vi "Audio Test.Calculate Freq Response.vi"(6 "Sweep Attribues":T1={"ReSampl Times(s)"=array[167426 elements], "Meas Phases (rad)"=[36.81553890925539, 8354.100868622301, 14959.386062088855, 20206.61147531608, 24374.996904709846, 27686.354004414785, 30316.88948878321, 32406.58165059181, 34066.62894449532, 35385.36721306204, 36432.970271774815, 37265.1840554823, 37926.29303158248, 38451.476685983085, 38868.681536741446, 39200.10824052903, 39463.39295419466, 39672.5458075507, 39838.69641775387, 39970.68613219857, 40075.5384988172, 40158.83301016359, 40225.00200445678, 40277.566521725035, 40319.32366977219, 40352.49546510379, 40378.84707330696, 40399.780738497255], "Meas Freqs (Hz)"=[20000.0, 15887.960215532483, 12621.363990517146, 10026.386447354535, 7964.941449056137, 6327.333643082476, 5026.421259584723, 3992.979049939437, 3172.0146143446227, 2519.8420997897483, 2001.7575515441654, 1590.1922170037706, 1263.2455339402636, 1003.5197392845996, 797.1940846627623, 633.28939505899, 503.08383568079324, 399.6487983186957, 317.48021039364005, 252.20564759765148, 200.35166475820458, 159.15896393970277, 126.4355643509683, 100.44016081182906, 79.78946395100115, 63.384591443608464, 50.35259335669159, 40.0], "Samples/rev"=26}, 8 "error in":errorcluster, 9 "Sine Sweep Params":T2={"Duration(s)"=2.0, "Amplitude"=1.0, "Freq Start"=20.0, "Freq End"=20000.0, "Samples/Sec"=44100.0} {"Amplitude" min=0.0 max=1.0 step=0.1}) -> (0 "error out":errorcluster, 2 "THD":cluster{"frequency":dbl[], "THD":dbl[]}(graph), 3 "Magnitude":cluster{"frequency":dbl[], "magnitude":dbl[]}(graph), 10 "Measured":waveform(dbl)(graph)={"t0"=timestamp(0 s since 1904-01-01), "dt"=2.2675736961451248e-05, "Y"=array[88200 elements]}, 11 "Stimulus":waveform(dbl)(graph)={"t0"=timestamp(0 s since 1904-01-01), "dt"=2.2675736961451248e-05, "Y"=array[88200 elements]})   [LabVIEW 2018]
uses:
  TypeDefs/AudioTest.Config, Sine Sweep Params.ctl
  TypeDefs/AudioTest.Sweep Attributes.ctl
  <vilib>/Utility/error.llb/DialogType.ctl
  <vilib>/addons/_NISVFA/_Shared subVIs/Controls/svc_Window.ctl
  <vilib>/addons/_NISVFA/_Shared subVIs/Common/svc_Get Waveform Subset (Index).vi
  <vilib>/addons/_NISVFA/_Shared subVIs/Common/svc_Get Array Subset (Index).vi
  <vilib>/addons/_NISVFA/_Shared subVIs/Common/svc_Coerce Index and Length.vi
  <vilib>/addons/_NISVFA/_Shared subVIs/Common/svc_Conditional Merge Error.vi
  <vilib>/Waveform/WDTOps.llb/WDT Copy Waveform dt DBL.vi
  <vilib>/measure/maresamp.llb/Align N Waveforms (single shot).vi
  <vilib>/addons/_NISVFA/_Baseband FFT/SVFA FFT Spectrum (Complex) (1 Ch).vi
  <vilib>/addons/Sound and Vibration/svt_Single Tone Measurements/SVT Gain and Phase (Frequency).vi
  <vilib>/addons/Sound and Vibration/svt_Distortion/SVT THD and Harmonic Components (Frequency) (1 Ch).vi
  Program Files (x86)/National Instruments/LabVIEW 2018/examples/Sound and Vibration/SoundVib_Audio Examples.lvlib
  <vilib>/measure/NI_MAPro.lvlib
  <vilib>/addons/Sound and Vibration/svt_Single Tone Measurements/SoundVib_SingleTone.lvlib
  <vilib>/addons/Sound and Vibration/svt_Continuous Swept Sine/SoundVib_ContSweptSine.lvlib
  <vilib>/addons/Sound and Vibration/svt_Distortion/SoundVib_Distortion.lvlib
panel:
  in  "Record":path
  in  "Sweep":path
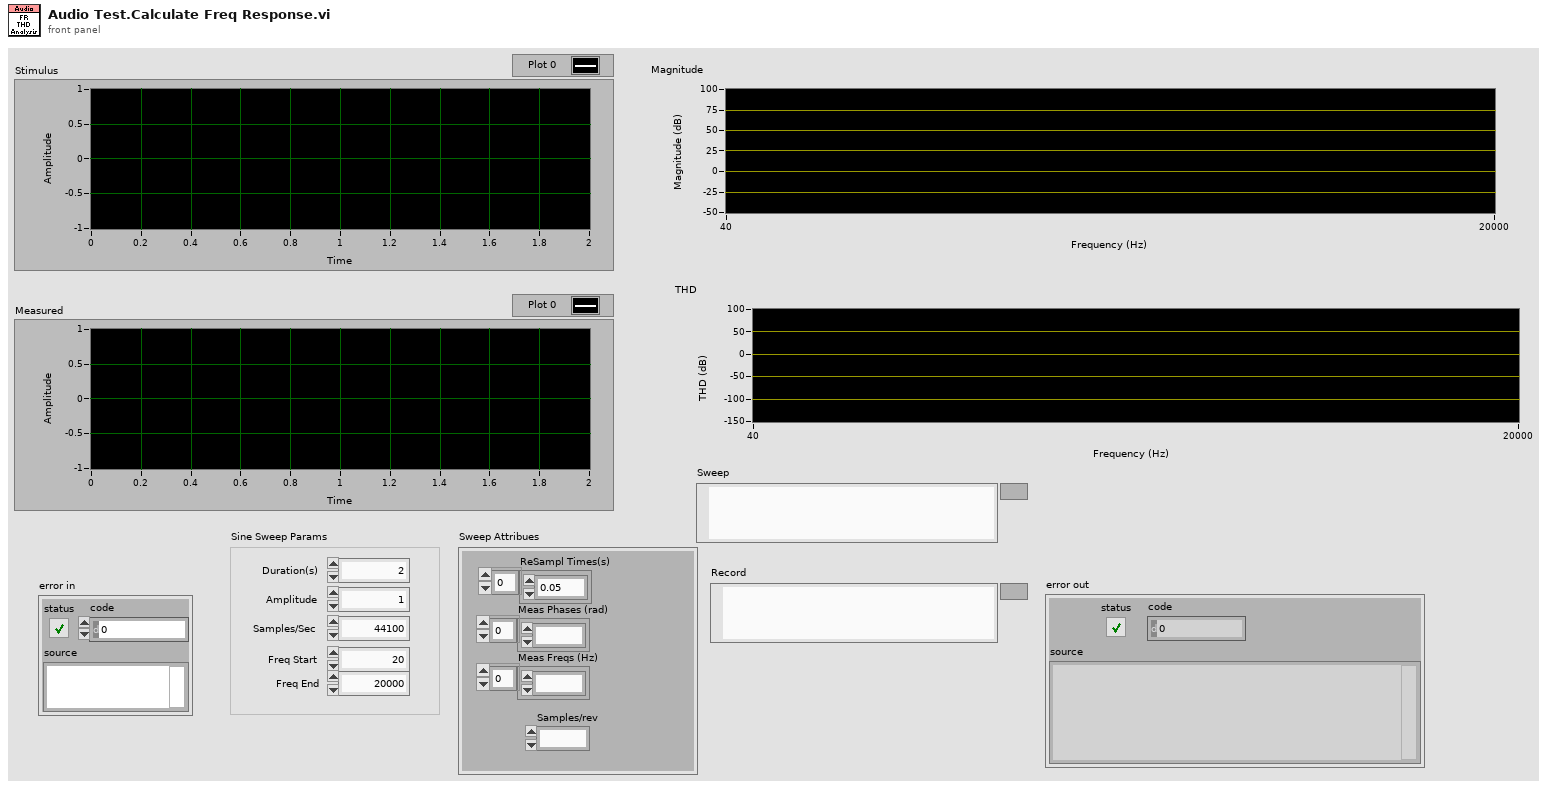
[diagram p1: front panel]
types:
  T1 = typedef "AudioTest.Sweep Attributes.ctl" = cluster{"ReSampl Times(s)":dbl[], "Meas Phases (rad)":dbl[], "Meas Freqs (Hz)":dbl[], "Samples/rev":i32}
  T2 = typedef "AudioTest.Config, Sine Sweep Params.ctl" = cluster{"Duration(s)":dbl, "Amplitude":dbl, "Freq Start":dbl, "Freq End":dbl, "Samples/Sec":dbl}
  T3 = typedef "DialogType.ctl" = u16
  T4 = cluster{"averaging mode":enum16{"No averaging", "Vector averaging", "RMS averaging", "Peak hold"}, "weighting mode":enum16{"Linear", "Exponential"}, "number of averages":u32, "linear mode":enum16{"One shot", "Auto restart"}}
  T5 = typedef "svc_Window.ctl" = u32
  T6 = typedef "svc_Spectrum Info.ctl" = cluster{"channel name":string, "description":string, "x-axis units":T7, "spectral info":cluster{"spectrum type":T8, "linear/dB":enum16{"linear", "dB"}, "window":u16, "window size":i32, "FFT size":i32}, "engineering units":T9, "custom label":string, "dB reference [EU]":dbl, "peak units":enum16{"rms", "peak", "peak-peak"}, "weighting filter":T10, "spectral density?":bool, "unit label":string, "spectrum skewed?":bool, "complimentary spectrum units":T11}
  T7 = typedef "svc_X-Axis Units.ctl" = u16
  T8 = typedef "svc_Spectrum Type.ctl" = enum16{"FFT Spectrum [complex]", "Amplitude [Magnitude]", "Power [Magnitude^2]", "Cross Spectrum [complex]", "Frequency Response [Complex]"}
  T9 = typedef "svc_Engineering Units Text Ring.ctl" = u16
  T10 = typedef "svc_Weighting Filter Text Ring.ctl" = u16
  T11 = typedef "svc_Complimentary Spectrum Units.ctl" = enum16{"none", "radians", "degrees", "cycles", "imaginary"}
  T12 = cluster{"complex spectrum response":cluster{"f0":dbl, "df":dbl, "complex spectrum":cdb[]}, "spectrum info":T6}
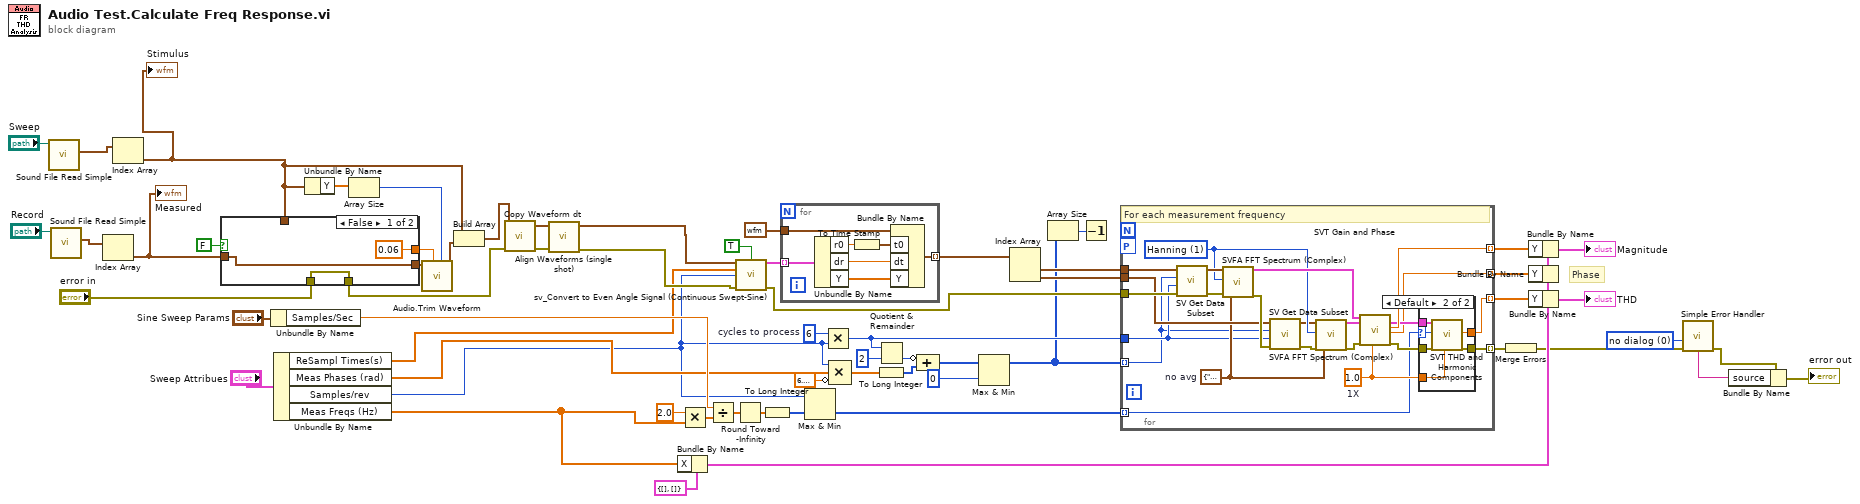
[diagram p0: block diagram]
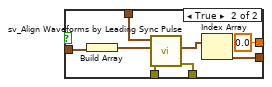
[diagram p2: hidden frame]
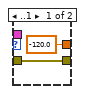
[diagram p3: hidden frame]
diagram:
  w25 = T3 0 items=["no dialog", "OK message", "continue or stop message", "OK message + warnings", "continue/stop + warnings"] ("type of dialog (OK msg:1)")
  w43 = 6  # cycles to process
  # "Phase"
  n1 = call <vilib>:"Sound File Read Simple.vi"("path"="Sweep") -> ("data"=w6:waveform(dbl)[])  [unwired: 7 in, 3 out]
  n2 = call <vilib>:"Sound File Read Simple.vi"("path"="Record") -> ("data"=w5:waveform(dbl)[])  [unwired: 7 in, 3 out]
  n3 = Index Array(array=w5) -> (element=w4:waveform(dbl))  [unwired: 1 in]
  "Measured" <- w4
  n4 = Index Array(array=w6) -> (element=w3:waveform(dbl))  [unwired: 1 in]
  "Stimulus" <- w3
  n5 = case shown="False" FALSE {
    tunnel: [w66 w73] -> w63
    tunnel: [w65 w71] -> w15
    tunnel: "error in" -> [w65 w70]
    tunnel: w4 -> [w66 w69]
    tunnel: w3 -> [_ w68]
    tunnel: [0.06 ("Max Delay") 0.0 ("Max Delay")] -> w1
    frame False {
    }
    frame True {
      n6 = Build Array(w69) -> (w72:waveform(dbl)[])
      n7 = call "sv_Align Waveforms by Leading Sync Pulse.vi"("error in (no error)"=w70, "response signals"=w72, "alignment reference signal"=w68) -> ("error out"=w71:errorcluster, "aligned signals"=w74:waveform(dbl)[])  [unwired: 4 in, 3 out]
      n8 = Index Array(array=w74) -> (element=w73:waveform(dbl))  [unwired: 1 in]
    }
  }
  n9 = Unbundle By Name("Sine Sweep Params") -> ("Samples/Sec"=w21:dbl)
  n10 = Unbundle By Name("Sweep Attribues") -> ("ReSampl Times(s)"=w19:dbl[], "Meas Phases (rad)"=w18:dbl[], "Samples/rev"=w17:i32, "Meas Freqs (Hz)"=w16:dbl[])
  n11 = Unbundle By Name(w3) -> ("Y"=w58:dbl[])
  n12 = Array Size(array=w58) -> (size(s)=w57:i32)
  n13 = call "Audio.Trim Waveform.vi"("Len"=w57, "Max Delay"=w1, "Data In"=w63) -> ("Data Out"=w62:waveform(dbl))  [unwired: 8 in]
  n14 = Build Array(w3, w62) -> (w59:waveform(dbl)[])
  n15 = call-poly <vilib>:"Copy Waveform dt.vi"("error in (no error)"=w15, "waveforms in"=w59) -> ("error out"=w60:errorcluster, "waveforms out"=w61:waveform(dbl)[])  [unwired: 8 in]
  n16 = call-poly <vilib>:"Align Waveforms (single shot).vi"("error in (no error)"=w60, "waveforms in"=w61) -> ("error out"=w22:errorcluster, "aligned waveforms out"=w23:waveform(dbl)[])  [unwired: 8 in]
  n17 = Bundle By Name(cluster=cluster{"X":dbl[], "Y":dbl[]} {"X"=[], "Y"=[]} ("THD vs Amplitude"), "X"=w16) -> (w54:cluster{"X":dbl[], "Y":dbl[]})
  n18 = Multiply(x=2.0 ("y"), y=w16) -> (x*y=w35:dbl[])
  n19 = Divide(x=w21, y=w35) -> (x/y=w34:dbl[])
  n20 = Round Toward -Infinity(1:w34) -> (0:w33:dbl[])
  n21 = call <vilib>:"sv_Convert to Even Angle Signal (Continuous Swept-Sine).vi"("scaled signals [EU]"=w23, "reset? (F)"=TRUE, "new sample time [s]"=w19, "new samples/rev"=w17, "error in (no error)"=w22) -> ("even-angle signals"=w53:cluster{"r0":dbl, "dr":dbl, "Y":dbl[]}[], "error out"=w29:errorcluster)  [unwired: 6 in, 3 out]
  n22 = To Long Integer(number=w33) -> (32bit integer=w31:i32[])
  n23 = for {
    tunnel: w53 -> [w81] mode=indexing
    tunnel: waveform(dbl) {"t0"=timestamp(0 s since 1904-01-01), "dt"=1.0, "Y"=[]} ("waveform out") -> [w76]
    tunnel: [w75] -> w24 mode=indexing
    n24 = Unbundle By Name(w81) -> ("r0"=w80:dbl, "dr"=w78:dbl, "Y"=w77:dbl[])
    n25 = To Time Stamp(1:w80) -> (0:w79:timestamp)
    n26 = Bundle By Name(cluster=w76, "t0"=w79, "dt"=w78, "Y"=w77) -> (w75:waveform(dbl))
  }
  n27 = Max & Min(x=w17, y=w31) -> (min(x,y)=w30:i32[])  [unwired: 1 out]
  n28 = Multiply(x=w43, y=w17) -> (x*y=w41:i32)
  n29 = Compound Arithmetic op=MULTIPLY(w17, w18, invert 6.283185307179586) -> (w37:dbl[])
  n30 = To Long Integer(number=w37) -> (32bit integer=w40:i32[])
  n31 = Quotient & Remainder(x=w41, y=2 ("x")) -> (floor(x/y)=w42:i32)  [unwired: 1 out]
  n32 = Compound Arithmetic op=ADD(invert w42, w40) -> (w38:i32[])
  n33 = Max & Min(x=w38, y=0 ("x")) -> (max(x,y)=w28:i32[])  [unwired: 1 out]
  n34 = Index Array(array=w24) -> (element #1=w49:waveform(dbl), element #2=w48:waveform(dbl))  [unwired: 2 in]
  n35 = Array Size(array=w28) -> (size(s)=w27:i32)
  n36 = Decrement(x=w27) -> ()  [unwired: 1 out]
  n37 = for {
    tunnel: w29 -> [w104]
    tunnel: [w98] -> w50 mode=indexing
    tunnel: [w97] -> w47 mode=indexing
    tunnel: w49 -> [w96]
    tunnel: w48 -> [w95]
    tunnel: [w87] -> w45 mode=indexing
    tunnel: [w86] -> w46 mode=indexing
    tunnel: w41 -> [w85]
    tunnel: w28 -> [w84] mode=indexing
    tunnel: w30 -> [w82] mode=indexing
    workers-P: _ -> [_]
    w83 = 1.0  # 1X
    w88 = T4 {"averaging mode"=enum."No averaging", "weighting mode"=enum."Exponential", "number of averages"=10, "linear mode"=enum."One shot"}  # no avg
    w99 = T5 1 items=["None"=0, "Hanning"=1, "Hamming"=2, "Blackman-Harris"=3, "Exact Blackman"=4, "Blackman"=5, "Flat Top"=6, "4 Term B-Harris "=7, "7 Term B-Harris"=8, "Low Sidelobe"=9, "Force"=64, "Exponential"=65, "Blackman Nuttall"=11, "Triangle"=30, "Bartlett-Hanning"=31, "Bohman"=32, "Parzen"=33, "Welch"=34, "Kaiser"=60, "Dolph-Chebyshev"=61, "Gaussian"=62] ("window")
    # "For each measurement frequency"
    n38 = call-poly <vilib>:"SV Get Data Subset.vi"("error in (no error)"=w104, "length (-1 = all)"=w85, "start index (0)"=w84, "waveform in"=w96) -> ("error out"=w102:errorcluster, "waveform subset"=w103:waveform(dbl))  [unwired: 2 in, 4 out]
    n39 = call-poly <vilib>:"SVFA FFT Spectrum (Complex).vi"("scaled signal [EU]"=w103, "window"=w99, "error in"=w102, "averaging parameters"=w88) -> ("complex spectrum"=w100:T12, "error out"=w101:errorcluster)  [unwired: 12 in, 2 out]
    n40 = call-poly <vilib>:"SV Get Data Subset.vi"("error in (no error)"=w101, "length (-1 = all)"=w85, "start index (0)"=w84, "waveform in"=w95) -> ("error out"=w93:errorcluster, "waveform subset"=w94:waveform(dbl))  [unwired: 2 in, 4 out]
    n41 = call-poly <vilib>:"SVFA FFT Spectrum (Complex).vi"("scaled signal [EU]"=w94, "window"=w99, "error in"=w93, "averaging parameters"=w88) -> ("complex spectrum"=w90:T12, "error out"=w89:errorcluster)  [unwired: 12 in, 2 out]
    n42 = call-poly <vilib>:"SVT Gain and Phase.vi"("complex spectrum\nstimulus X"=w100, "complex spectrum\nresponse Y"=w90, "error in (no error)"=w89, "expected fundamental frequency [Hz]"=w83) -> ("dup complex spectrum\nresponse Y"=w92:T12, "gain"=w97:dbl, "phase lag"=w86:dbl, "error out"=w91:errorcluster)  [unwired: 8 in, 4 out]
    n43 = case shown="Default" w82 {
      selector: w82 -> [_ w107]
      tunnel: [w106 w112] -> w98
      tunnel: w92 -> [_ w111]
      tunnel: w91 -> [w106 w110]
      tunnel: [-120.0 ("THD") w109] -> w87
      tunnel: w83 -> [_ w108]
      frame ..1 {
      }
      frame Default {
        n44 = call-poly <vilib>:"SVT THD and Harmonic Components.vi"("complex spectrum"=w111, "maximum harmonic"=w107, "error in (no error)"=w110, "expected fundamental frequency [Hz]"=w108) -> ("THD"=w109:dbl, "error out"=w112:errorcluster)  [unwired: 8 in, 6 out]
      }
    }
  }
  n45 = Merge Errors(w50) -> (w26:errorcluster)
  n46 = Bundle By Name(cluster=w54, "Y"=w47) -> (→"Magnitude":cluster{"X":dbl[], "Y":dbl[]})
  n47 = Bundle By Name(cluster=w54, "Y"=w46) -> ()  [unwired: 1 out]
  n48 = Bundle By Name(cluster=w54, "Y"=w45) -> (→"THD":cluster{"X":dbl[], "Y":dbl[]})
  n49 = call <vilib>:"Simple Error Handler.vi"("type of dialog (OK msg:1)"=w25, "error in (no error)"=w26) -> ("error out"=w11:errorcluster, "message"=w13:string)  [unwired: 3 in, 3 out]
  n50 = Bundle By Name(cluster=w11, "source"=w13) -> (→"error out":errorcluster)
